vi "ExposeMapperGetValueNameFromVariant.vi"(11 "Data Val Ref in":refnum<data-value>) -> (1 "System Type":T1, 3 "Name":string)   [LabVIEW 2017]
uses:
  <vilib>/Utility/Data Type/Type Definitions/Data Type.ctl
  <vilib>/Utility/Data Type/NI_Data Type.lvlib
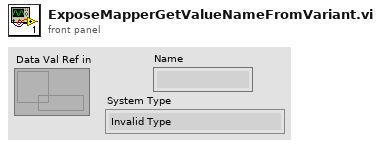
[diagram p1: front panel]
types:
  T1 = typedef "NI_Data Type.lvlib/Data Type.ctl" = enum8{"Invalid Type", "Void", "I8", "I16", "I32", "I64", "U8", "U16", "U32", "U64", "Single Float", "Double Float", "Extended Float", "Single Complex", "Double Complex", "Extended Complex", "Enum U8", "Enum U16", "Enum U32", "Enum U64", "Single Float With Unit", "Double Float With Unit", "Extended Float With Unit", "Single Complex with Unit", "Double Complex with Unit", "Extended Complex with Unit", "Boolean", "String", "Path", "Picture", "Tag", "Array", "Cluster", "Variant", "LV Variant", "Waveform", "Timestamp", "Digital Waveform", "Digital Data", "ExpressData", "Refnum", "External Data", "VI", "Poly VI", "LabVIEW Class Instance", "Fixed Point"}
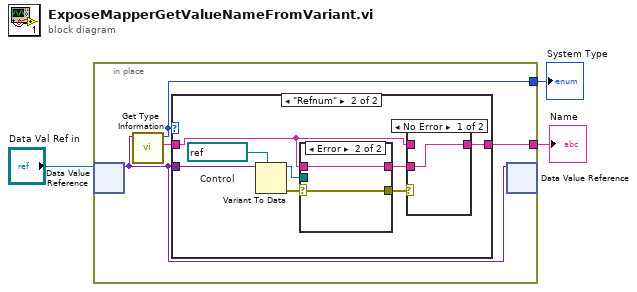
[diagram p0: block diagram]
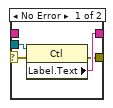
[diagram p4: hidden frame]
diagram:
  n1 = in-place {
    in-place-border: [w6] -> w3
    in-place-border: [w4] -> w1
    n2 = in-place-dvr #1("Data Val Ref in") -> (w5:variant)  [unwired: 1 out]
    n3 = call <vilib>:"Get Type Information.vi"("Variant"=w5) -> ("Name"=w7:string, "Type"=w4:T1)  [unwired: 6 in, 3 out]
    n4 = case shown="\"Refnum\"" w4 {
      tunnel: w7 -> [w8 w11]
      tunnel: [w8 w10] -> w6
      tunnel: w5 -> [_ w9]
      frame Default {
      }
      frame "Refnum" {
        w16 = refnum<vi> refnum  # Control
        n5 = Variant To Data(type=w16, Variant=w9) -> (data=w14:refnum<vi>, error out=w15:errorcluster)  [unwired: 1 in]
        n6 = case shown="Error" w15 {
          selector: w15 -> [w20 w23]
          tunnel: w11 -> [_ w24]
          tunnel: [w21 w24] -> w12
          tunnel: w14 -> [w22 _]
          tunnel: [w19 w23] -> w13
          frame No Error {
            n7 = property class="Ctl"(reference=w22, error in=w20) -> (error out=w19:errorcluster, "Label.Text"=w21:string)  [unwired: 1 out]
          }
          frame Error {
          }
        }
        n8 = case shown="No Error" w13 {
          tunnel: w12 -> [w17 _]
          tunnel: w11 -> [_ w18]
          tunnel: [w17 w18] -> w10
          frame No Error {
          }
          frame Error {
          }
        }
      }
    }
    n9 = in-place-dvr #1(w5) -> ()  [unwired: 2 out]
  }
  "Name" <- w3
  "System Type" <- w1
